vi "CMD Only (FPGA).vi"() -> ()   [LabVIEW 2019]
uses:
  <vilib>/eio/EIONode/EIONode.xnode
  <vilib>/rvi/eio/common/nirviEmuTemplateMethod_errors.vi
panel:
  in  "PWM Period (Ticks)":u32=40000000
  in  "Duty (Ticks) 1":i32
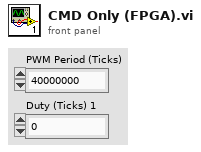
[diagram p1: front panel]
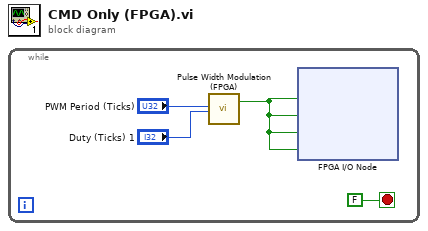
[diagram p0: block diagram]
diagram:
  n1 = while {
    stop <- FALSE stop-if-true
    n2 = call "Pulse Width Modulation (FPGA).vi"("PWM Period (Ticks)"="PWM Period (Ticks)", "PWM Duty Cycle (Ticks)"="Duty (Ticks) 1") -> ("PWM DO"=w1:bool)  [unwired: 14 in, 3 out]
    n3 = xnode "FPGA I/O Node"("RMC/DIO0"=w1, "RMC/DIO1"=w1, "RMC/DIO2"=w1, "RMC/DIO3"=w1) -> ()  [unwired: 5 in, 5 out]
  }
